vi "mmWave Test Main.vi"() -> ()   [LabVIEW 2019]
doc: "Simple Qued Message Handler type of state machine.\nAlways use this template if the VI is a UI used by a user and it is more complex than a dialog.\n(Unless you're usig something more advanced like Actor Framework)\n\nBolder Software LLC"
uses:
  Support/MessageAPI/RunTest.ctl
  Classes/aparCfg/aparCfg.lvclass
  Classes/Sequence/Sequence.lvclass
  Classes/ExecutionControls/ExecutionControls.lvclass
  Classes/ExecutionStatus/ExecutionStatus.lvclass
  Classes/UI MotionStatus/UI MotionStatus.lvclass
  Classes/SendMessage/SendMessage.lvclass
  Classes/UI ExecutionCtrls/UI ExecutionCtrls.lvclass
  Classes/UI MotionStatus/MotionStatusLEDCtrlRefs.ctl
  Classes/UI MotionStatus/PositonIndicatorsCtrlRefs.ctl
  Classes/UI ExecutionCtrls/MotionExecutionCtrlRefs.ctl
  Classes/UI ExecutionCtrls/mmWaveMotionCrtlRefs.ctl
  Classes/ExecutionControls/ExecutionCtrlRefs.ctl
  Classes/Datalog/DatalogSubvis/SearchableTag.ctl
  Classes/Sequence/SequenceSubvis/RF Direction.ctl
  Classes/Sequence/SequenceSubvis/PolarizationSelect.ctl
  APARMainSubvis/VXM Public API/singleAxisMoveDef.ctl
  APARMainSubvis/VXM Public API/mmWaveAxis.ctl
  Support/MessageQue/MessageQue.lvlib
  Support/UserEvent-ExitEventLoop/UserEvent-ExitEventLoop.lvlib
  Classes/VXMCfg/VXMCfg.lvclass
  Classes/Datalog/DataLog.lvclass
panel:
  out "UIM EventCode":i32
  out "UIM Numeric":dbl
  out "RT2 moving":bool
  out "RT1 moving":bool
  out "BS4 moving":bool
  out "RT2":sgl caption="RT 2, degrees" format="%.2f"
  out "RT1":sgl caption="RT1, degrees" format="%.2f"
  out "BS4":sgl caption="BS 4, mm" format="%.2f"
  in  "Module, 0-63":dbl min=0.0 max=63.0 step=1.0
  out "Temperature, °C":dbl format="%.1g"
  in  "ac read temp":bool
  in  "ac reset":bool
  in  "One Sweep":bool
  in  "Stop Motion":bool
  out "SubSystem 3":bool
  out "SubSystem 2":bool
  in  "FindHomeAll":bool
  in  "Raster Test Sequence Start":bool
  in  "P&M Test Sequence Start":bool
  in  "Run P&M Test":T1
  in  "Polarization":u16(ring) items=["Vertical", "Horizontal"]
  in  "Move to Pos.":bool
  in  "Position":i32=1 caption="Antenna\nPosition" min=0 max=63 step=1
  in  "SeqPanel":bool
  in  "Data File Name":string
  in  "Merge Results":bool
  in  "Merge File and Path":path
  out "Antenna/Raster\nPosition":string
  out "SubSystem 1":bool
  out "RT3 moving":bool
  out "BS3 moving":bool
  out "BS2 moving":bool
  out "BS1 moving":bool
  out "RT3":sgl caption="RT 3, degrees" format="%.2f"
  out "BS3":sgl caption="BS3, mm" format="%.2f"
  out "BS2":sgl caption="BS 2, mm" format="%.2f"
  out "BS1":sgl caption="BS1, mm" format="%.2f"
  in  "Tab":T2(tab)
  in  "Run mode 2":bool
  in  "Run mode 1":bool
  in  "Decimate Update":i32=1
  out "Agilent N5222A Traces":T3(graph)
  out "Progress":u8(slide) scale=0.0..100.0
  out "Sequence Status":string
  in  "ConfigPanel":bool
  in  "Stop":bool
  in  "Run Mode 3":bool
  in  "Pause":bool
  in  "AO Board 2 voltages":dbl[](array[numeric])
  in  "AO Board 1 voltages":dbl[](array[numeric])
  in  "ac d cmd":bool
  in  "RT2 Home Button":bool
  in  "RT2 Jog Neg.":bool
  in  "RT2 Jog Pos.":bool
  in  "Set RT2 Position, Deg.":dbl format="%.4f"
  in  "BS4 Home Button":bool
  in  "BS4 Jog Neg.":bool
  in  "BS4 Jog Pos.":bool
  in  "Set BS4 Position, mm":dbl format="%.4f"
  in  "BS3 Home Button":bool
  in  "BS3 Jog Neg.":bool
  in  "BS3 Jog Pos.":bool
  in  "Set BS3 Position, mm":dbl format="%.4f"
  in  "setHomeSS2":bool
  in  "setHomeSS1":bool
  in  "T Home Button":bool
  in  "T Jog Neg.":bool
  in  "T Jog Pos.":bool
  in  "Set RT3 Position, Deg.":dbl format="%.4f"
  in  "Z Home Button":bool
  in  "Z Jog Neg.":bool
  in  "Z Jog Pos.":bool
  in  "Set RT1 Position, Deg":dbl format="%.4f"
  in  "Y Home Button":bool
  in  "Y Jog Neg.":bool
  in  "Y Jog Pos.":bool
  in  "Set BS2 Position, mm":dbl format="%.4f"
  in  "X Home Button":bool
  in  "X Jog Neg.":bool
  in  "X Jog Pos.":bool
  in  "Set BS1 Position, mm":dbl format="%.4f"
  in  "HomeAll":bool
  in  "MoveAllAbsolute":bool
  in  "Generate \"DAQ\" Loop TestError":bool
  in  "test error":errorcluster
  in  "Generate \"Main\" Loop TestError":bool
  out "i event":i32=6 caption="ievent"
  out "Command":string
  out "i main":i32=6
  # "Park and Measure Positions"
  # "<< make subsyst 1, add button for subsyst 2"
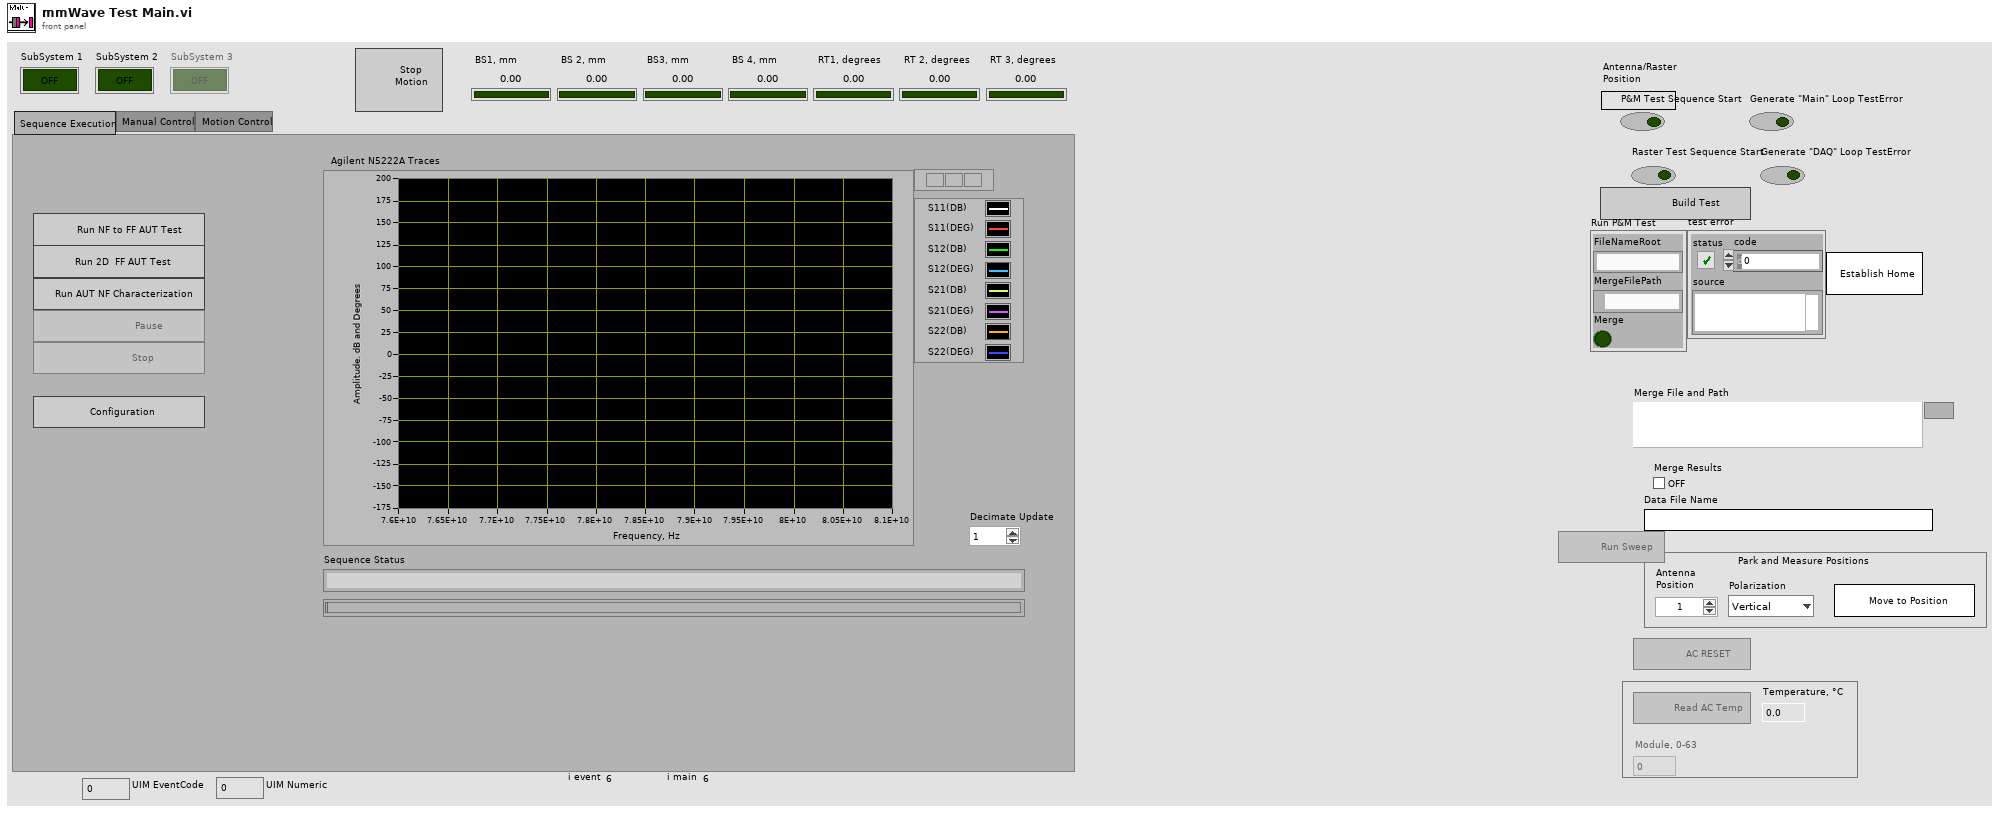
[diagram p1: front panel]
types:
  T1 = typedef "RunTest.ctl" = cluster{"FileNameRoot":string, "MergeFilePath":path, "Merge":bool}
  T2 = enum32{"Sequence Execution", "Manual Control", "Motion Control"}
  T3 = cluster{"array type (2D Dbl)":dbl[], "array type (2D Dbl)":dbl[]}[]
  T4 = cluster{"aparCfg":refnum<class "aparCfg.lvclass">, "Sequence":refnum<class "Sequence.lvclass">, "ExecCtrls":refnum<class "ExecutionControls.lvclass">, "ExecStatus":refnum<class "ExecutionStatus.lvclass">, "graph":i32, "MotionStatus":refnum<class "UI MotionStatus.lvclass">, "SendUIMsg":refnum<class "SendMessage.lvclass">, "MotionExecCtrls":refnum<class "UI ExecutionCtrls.lvclass">}
  T5 = typedef "MultipleMessageQues vxm.ctl" = cluster{"Main que":T6, "Error que":T6, "VXM Svc que":T6, "Listener que":T6, "VXM ACK que":T6, "DAQ que":T6, "Alignment que":T6}
  T6 = typedef "MessageQue.lvlib/MessageQue.ctl" = refnum<queue>
  T7 = typedef "DataLog.lvclass/SearchableTag.ctl" = cluster{"Module, 0-63":i32, "RF Direction Tx0":T8, "Polarization, V0 H1":T9, "AO-64 Array":dbl[]}
  T8 = typedef "RF Direction.ctl" = enum16{"Tx - RF In", "Rx - RF Out"}
  T9 = typedef "PolarizationSelect.ctl" = enum16{"Vertical", "Horizontal"}
  T10 = typedef "mmWaveAxis.ctl" = string
  T11 = typedef "singleAxisMoveDef.ctl" = cluster{"mmWave Axis":T10, "eng. value":dbl}
  T12 = cluster{"Move Type":string, "Positions":T11[], "Position (Antenna or Raster)":i32, "Polarization":u16}
  T13 = typedef "MotionExecutionCtrlRefs.ctl" = cluster{"MoveAllAbsolute":refnum<vi>, "Move to Pos.":refnum<vi>, "HomeAll":refnum<vi>, "FindHomeAll":refnum<vi>, "X Jog Pos.":refnum<vi>, "X Jog Neg.":refnum<vi>, "Y Jog Pos.":refnum<vi>, "Y Jog Neg. ":refnum<vi>, "Z Jog Pos.":refnum<vi>, "Z Jog Neg.":refnum<vi>, "T Jog Pos.":refnum<vi>, "T Jog Neg.":refnum<vi>, "X Home Button":refnum<vi>, "Y Home Button":refnum<vi>, "Z Home Button":refnum<vi>, "T Home Button":refnum<vi>}
  T14 = typedef "PositonIndicatorsCtrlRefs.ctl" = cluster{"BS1":refnum<vi>, "BS2":refnum<vi>, "BS3":refnum<vi>, "BS4":refnum<vi>, "RT3":refnum<vi>, "RT2":refnum<vi>, "RT1":refnum<vi>}
  T15 = typedef "MotionStatusLEDCtrlRefs.ctl" = cluster{"BS1":refnum<vi>, "BS2":refnum<vi>, "BS3":refnum<vi>, "BS4":refnum<vi>, "RT1":refnum<vi>, "RT2":refnum<vi>, "RT3":refnum<vi>}
  T16 = typedef "mmWaveMotionCrtlRefs.ctl" = cluster{"BS3 Jog Neg. 2":refnum<vi>, "BS3 Jog Pos. 2":refnum<vi>, "BS3 Home Button 2":refnum<vi>, "BS4 Jog Neg. 2":refnum<vi>, "BS4 Jog Pos. 2":refnum<vi>, "BS4 Home Button 2":refnum<vi>, "RT2 Jog Neg. 2":refnum<vi>, "RT2 Jog Pos. 2":refnum<vi>, "RT2 Home Button 2":refnum<vi>}
  T17 = typedef "ExecutionCtrlRefs.ctl" = cluster{"Tab":refnum<vi>, "BuildSeqDlg":refnum<vi>, "Run":refnum<vi>, "Pause":refnum<vi>, "Stop":refnum<vi>, "ConfigPanel":refnum<vi>, "SeqStatus":refnum<vi>, "Run raster":refnum<vi>}
  T18 = cluster{"mmWave Names":string[], "Positions this subsystem":dbl[]}
  T19 = typedef "seqConfig.ctl" = cluster{"TempXMLFilePath":path, "Motion":bool}
  T20 = typedef "ACConfig.ctl" = cluster{"Board 1 alias":string, "Board 1 Enable":bool, "Board 2 alias":string, "Board 2 Enable":bool}
  T21 = typedef "N5222AConfig.ctl" = cluster{"ResourceName":string, "Enable":bool, "Channel":i32, "CalFileName":string, "MeasName":string, "TempDatFile":string, "Power, dBm":dbl, "NumPoints":i32, "Start Freq, Hz":dbl, "Stop Freq, Hz":dbl, "NumAverages":i32, "Sweep Type":i32, "IF Bandwidth":dbl}
  T22 = typedef "Mode1TestProperties.ctl" = cluster{"Probe Horizontal Polarization":bool, "Probe Vertical Polarization":bool, "Data File Name":string, "RF In/Out of antenna":T8, "Raster XY Points":cluster{"X mm":dbl, "Y mm":dbl}[]}
  T23 = typedef "Mode2TestProperties.ctl" = cluster{"Probe Horizontal Polarization":bool, "Probe Vertical Polarization":bool, "Upload TR Module file":path, "Data File Name":string, "RF In/Out of antenna":T8, "RT3 Positions, degrees":dbl[]}
  T24 = typedef "Mode3TestProperties.ctl" = cluster{"Probe Horizontal Polarization":bool, "Probe Vertical Polarization":bool, "Upload TR Module file":path, "Data File Name":string, "RF In/Out of antenna":T8}
  T25 = typedef "UIMessage.ctl" = cluster{"EventCode":i32, "Numeric":dbl, "String":string, "Variant":variant}
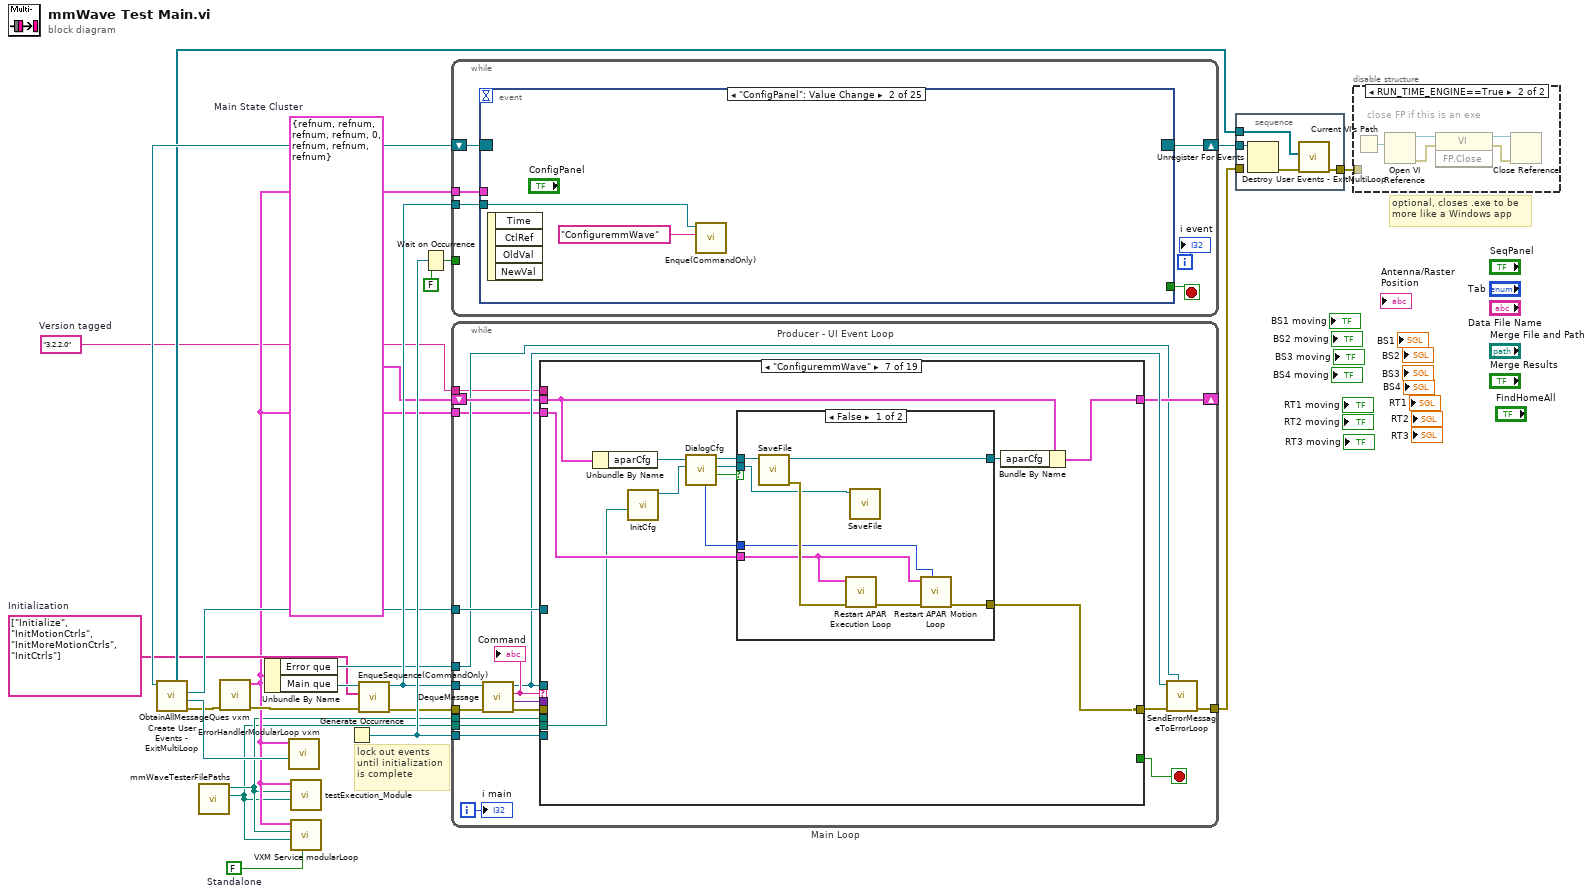
[diagram p0: block diagram]
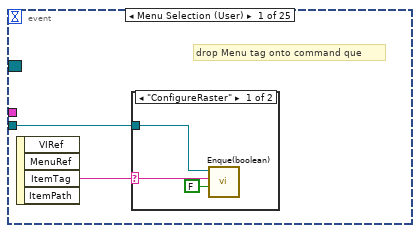
[diagram p3: hidden frame]
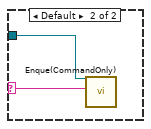
[diagram p4: hidden frame]
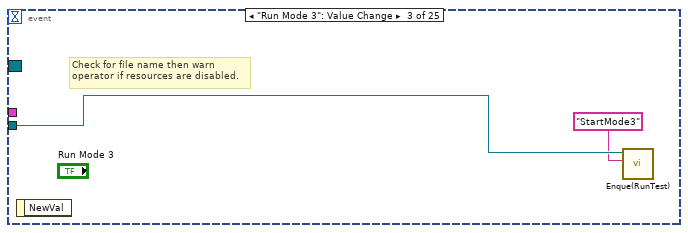
[diagram p5: hidden frame]
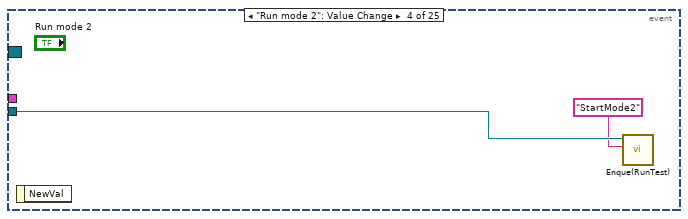
[diagram p6: hidden frame]
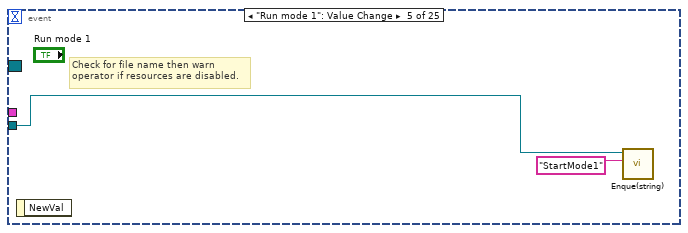
[diagram p7: hidden frame]
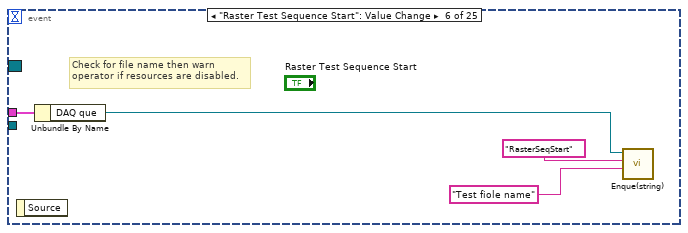
[diagram p8: hidden frame]
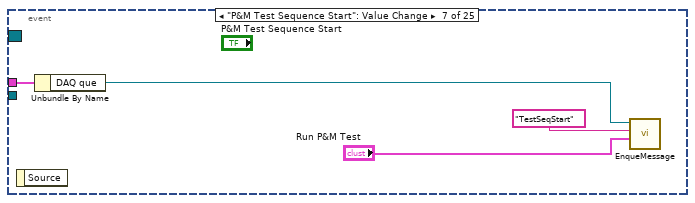
[diagram p9: hidden frame]
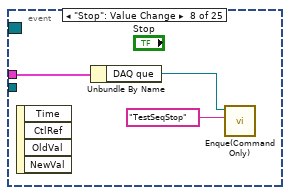
[diagram p10: hidden frame]
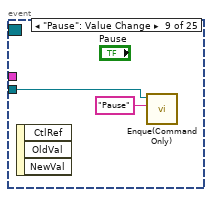
[diagram p11: hidden frame]
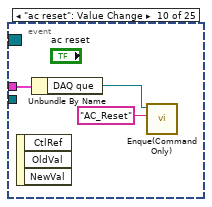
[diagram p12: hidden frame]
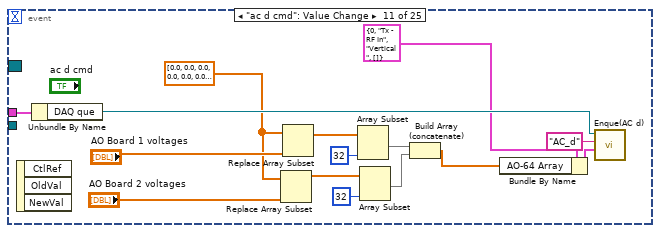
[diagram p13: hidden frame]
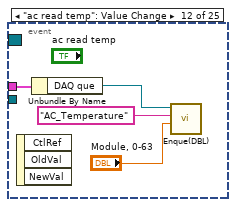
[diagram p14: hidden frame]
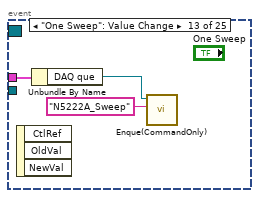
[diagram p15: hidden frame]
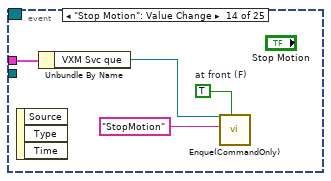
[diagram p16: hidden frame]
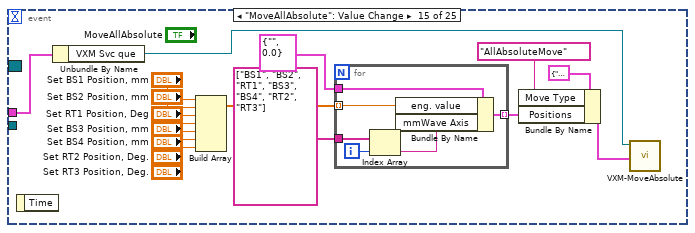
[diagram p17: hidden frame]
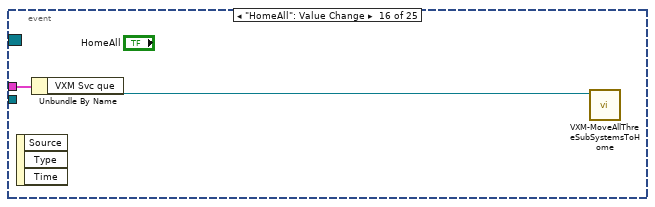
[diagram p18: hidden frame]
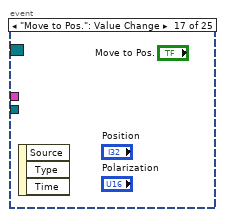
[diagram p19: hidden frame]
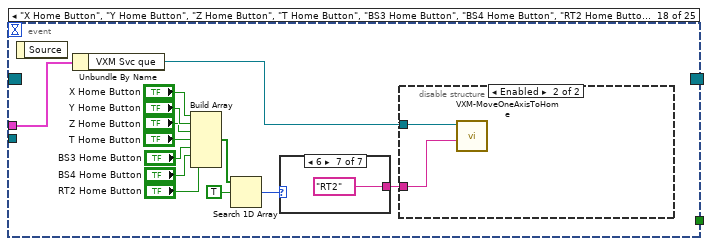
[diagram p20: hidden frame]
diagram:
  w2 = "3.2.2.0"  # Version tagged
  w3 = FALSE  # Standalone
  w9 = string[] ["Initialize", "InitMotionCtrls", "InitMoreMotionCtrls", "InitCtrls"]  # Initialization
  w15 = T4 {"aparCfg"=refnum, "Sequence"=refnum, "ExecCtrls"=refnum, "ExecStatus"=refnum, "graph"=0, "MotionStatus"=refnum, "SendUIMsg"=refnum, "MotionExecCtrls"=refnum}  # Main State Cluster
  # "lock out events\nuntil initialization\nis complete"
  # "optional, closes .exe to be \nmore like a Windows app"
  n1 = call "Create User Events - ExitMultiLoop.vi"() -> ("error out"=w7:errorcluster, "ExitALLLoops event out"=w8:refnum<user-event>, "ExitEventLoop event out"=w10:refnum<user-event>, "Events Registration Refnum"=w18:refnum<event-registration>, "user event array"=w11:refnum<user-event>[])  [unwired: 7 in]
  n2 = call "mmWaveTesterFilePaths.vi"() -> ("Config File Path Motion"=w1:path, "Config File Path"=w4:path)  [unwired: 6 in, 4 out]
  n3 = call "ObtainAllMessageQues vxm.vi"("error in"=w7) -> ("error out"=w6:errorcluster, "MessageQues"=w5:T5)  [unwired: 9 in]
  n4 = Unbundle By Name(w5) -> ("Error que"=w12:T6, "Main que"=w14:T6)
  n5 = call "ErrorHandlerModularLoop vxm.vi"("exit event source"=w8, "MessageQues"=w5) -> ()  [unwired: 9 in, 1 out]
  n6 = call "testExecution_Module.vi"("Motion Cfg File path"=w1, "Cfg File path"=w4, "MessageQues"=w5) -> ()  [unwired: 9 in]
  n7 = call "VXM Service modularLoop.vi"("Standalone"=w3, "Motion Cfg File path"=w1, "Cfg File path"=w4, "MessageQues"=w5) -> ()  [unwired: 8 in]
  n8 = Generate Occurrence() -> (w23:refnum<k4>)
  n9 = call "EnqueSequence(CommandOnly).vi"("error in"=w6, "Message Commands"=w9, "Message que"=w14) -> ("error out"=w20:errorcluster, "Message que out"=w19:T6)  [unwired: 7 in]
  n10 = Wait on Occurrence(1:FALSE ("ignore previous (T)"), 2:w23) -> (0:w17:bool)  [unwired: 1 in]
  n11 = while "Producer - UI Event Loop" {
    shift-right: [w25] -> w22
    shift-left: w18 -> [w26]
    tunnel: w19 -> [w28]
    tunnel: w17 -> [_]
    tunnel: w5 -> [w24]
    i -> [w29]
    stop <- w27 stop-if-true
    n12 = event shown="[1] \"ConfigPanel\": Value Change" {
      selector: w26 -> [_ _ _ _ _ _ _ _ _ _ _ _ _ _ _ _ _ _ _ _ _ _ _ _ _]
      dyn-events: [_ _ _ _ _ _ _ _ _ _ _ _ _ _ _ _ _ _ _ _ _ _ _ _ _] -> w25
      timeout: _ -> [_ _ _ _ _ _ _ _ _ _ _ _ _ _ _ _ _ _ _ _ _ _ _ _ _]
      tunnel: w28 -> [w31 w38 w40 w42 w43 _ _ _ w57 _ _ _ _ _ _ _ _ _ _ _ _ w208 w216 _ _]
      tunnel: [_ _ _ _ _ _ _ _ _ _ _ _ _ _ _ _ _ _ _ _ _ _ _ _ TRUE ("Discard?")] -> w27
      tunnel: w24 -> [_ _ _ _ _ w47 w52 w54 _ w59 w74 w78 w81 w83 w102 w110 _ w117 w147 w176 w200 w211 w214 w222 _]
      event Menu Selection (User) {
        # "drop Menu tag onto command que"
        n13 = event-data() -> ("ItemTag"=w30:string)  [unwired: 1 in, 3 out]
        n14 = case shown="\"ConfigureRaster\"" w30 {
          selector: w30 -> [w32 w35]
          tunnel: w31 -> [w34 w36]
          frame "ConfigureRaster" {
            n15 = call "Enque(boolean).vi"("Message Payload  Boolean"=FALSE, "Message Command"=w32, "Message que"=w34) -> ()  [unwired: 7 in, 2 out]
          }
          frame Default {
            n16 = call "Enque(CommandOnly).vi"("Message Command"=w35, "Message que"=w36) -> ()  [unwired: 8 in, 2 out]
          }
        }
      }
      event "ConfigPanel": Value Change {
        n17 = event-data() -> ()  [unwired: 1 in, 4 out]
        n18 = call "Enque(CommandOnly).vi"("Message Command"="ConfiguremmWave", "Message que"=w38) -> ()  [unwired: 8 in, 2 out]
      }
      event "Run Mode 3": Value Change {
        # "Check for file name then warn\noperator if resources are disabled."
        n19 = event-data() -> ()  [unwired: 1 in, 1 out]
        n20 = call "Enque(RunTest).vi"("Message Command"="StartMode3", "Message que"=w40) -> ()  [unwired: 8 in, 2 out]
      }
      event "Run mode 2": Value Change {
        n21 = event-data() -> ()  [unwired: 1 in, 1 out]
        n22 = call "Enque(RunTest).vi"("Message Command"="StartMode2", "Message que"=w42) -> ()  [unwired: 8 in, 2 out]
      }
      event "Run mode 1": Value Change {
        # "Check for file name then warn\noperator if resources are disabled."
        n23 = event-data() -> ()  [unwired: 1 in, 1 out]
        n24 = call "Enque(string).vi"("Message Command"="StartMode1", "Message que"=w43) -> ()  [unwired: 8 in, 2 out]
      }
      event "Raster Test Sequence Start": Value Change {
        # "Check for file name then warn\noperator if resources are disabled."
        n25 = event-data() -> ()  [unwired: 1 in, 1 out]
        n26 = Unbundle By Name(w47) -> ("DAQ que"=w46:T6)
        n27 = call "Enque(string).vi"("Message Payload string"="Test fiole name", "Message Command"="RasterSeqStart", "Message que"=w46) -> ()  [unwired: 7 in, 2 out]
      }
      event "P&M Test Sequence Start": Value Change {
        n28 = event-data() -> ()  [unwired: 1 in, 1 out]
        n29 = Unbundle By Name(w52) -> ("DAQ que"=w51:T6)
        n30 = call "EnqueMessage.vi"("Message Payload"="Run P&M Test", "Message Command"="TestSeqStart", "Message que"=w51) -> ()  [unwired: 7 in, 2 out]
      }
      event "Stop": Value Change {
        n31 = event-data() -> ()  [unwired: 1 in, 4 out]
        n32 = Unbundle By Name(w54) -> ("DAQ que"=w53:T6)
        n33 = call "Enque(CommandOnly).vi"("Message Command"="TestSeqStop", "Message que"=w53) -> ()  [unwired: 8 in, 2 out]
      }
      event "Pause": Value Change {
        n34 = event-data() -> ()  [unwired: 1 in, 3 out]
        n35 = call "Enque(CommandOnly).vi"("Message Command"="Pause", "Message que"=w57) -> ()  [unwired: 8 in, 2 out]
      }
      event "ac reset": Value Change {
        n36 = event-data() -> ()  [unwired: 1 in, 3 out]
        n37 = Unbundle By Name(w59) -> ("DAQ que"=w58:T6)
        n38 = call "Enque(CommandOnly).vi"("Message Command"="AC_Reset", "Message que"=w58) -> ()  [unwired: 8 in, 2 out]
      }
      event "ac d cmd": Value Change {
        w71 = dbl[] [0.0, 0.0, 0.0, 0.0, 0.0, 0.0, 0.0, 0.0, 0.0, 0.0, 0.0, 0.0, 0.0, 0.0, 0.0, 0.0, 0.0, 0.0, 0.0, 0.0, 0.0, 0.0, 0.0, 0.0, 0.0, 0.0, 0.0, 0.0, 0.0, 0.0, 0.0, 0.0] ("AO Board 1 voltages")
        n39 = event-data() -> ()  [unwired: 1 in, 3 out]
        n40 = Unbundle By Name(w74) -> ("DAQ que"=w73:T6)
        n41 = Replace Array Subset(array=w71, new element="AO Board 2 voltages") -> (w66:dbl[])  [unwired: 1 in]
        n42 = Replace Array Subset(array=w71, new element="AO Board 1 voltages") -> (w68:dbl[])  [unwired: 1 in]
        n43 = Array Subset(array=w68, length=32) -> (w65:dbl[])  [unwired: 1 in]
        n44 = Array Subset(array=w66, length=32) -> (w64:dbl[])  [unwired: 1 in]
        n45 = Build Array (concatenate)(w65, w64) -> (w61:dbl[])
        n46 = Bundle By Name(cluster=T7 {"Module, 0-63"=0, "RF Direction Tx0"=enum."Tx - RF In", "Polarization, V0 H1"=enum."Vertical", "AO-64 Array"=[]} ("d Cmd Payload"), "AO-64 Array"=w61) -> (w62:T7)
        n47 = call "Enque(AC d).vi"("d Cmd Payload"=w62, "Message Command"="AC_d", "Message que"=w73) -> ()  [unwired: 7 in, 2 out]
      }
      event "ac read temp": Value Change {
        n48 = event-data() -> ()  [unwired: 1 in, 3 out]
        n49 = Unbundle By Name(w78) -> ("DAQ que"=w77:T6)
        n50 = call "Enque(DBL).vi"("Message Payload DBL Numeric"="Module, 0-63", "Message Command"="AC_Temperature", "Message que"=w77) -> ()  [unwired: 7 in, 2 out]
      }
      event "One Sweep": Value Change {
        n51 = event-data() -> ()  [unwired: 1 in, 3 out]
        n52 = Unbundle By Name(w81) -> ("DAQ que"=w80:T6)
        n53 = call "Enque(CommandOnly).vi"("Message Command"="N5222A_Sweep", "Message que"=w80) -> ()  [unwired: 8 in, 2 out]
      }
      event "Stop Motion": Value Change {
        w86 = TRUE  # at front (F)
        n54 = event-data() -> ()  [unwired: 1 in, 3 out]
        n55 = Unbundle By Name(w83) -> ("VXM Svc que"=w84:T6)
        n56 = call "Enque(CommandOnly).vi"("at front (F)"=w86, "Message Command"="StopMotion", "Message que"=w84) -> ()  [unwired: 7 in, 2 out]
      }
      event "MoveAllAbsolute": Value Change {
        n57 = event-data() -> ()  [unwired: 1 in, 1 out]
        n58 = Unbundle By Name(w102) -> ("VXM Svc que"=w101:T6)
        n59 = Build Array("Set BS1 Position, mm", "Set BS2 Position, mm", "Set RT1 Position, Deg", "Set BS3 Position, mm", "Set BS4 Position, mm", "Set RT2 Position, Deg.", "Set RT3 Position, Deg.") -> (w89:dbl[])
        n60 = for {
          tunnel: T11 {"mmWave Axis"="", "eng. value"=0.0} ("Move") -> [w108]
          tunnel: w89 -> [w107] mode=indexing
          tunnel: [w106] -> w88 mode=indexing
          tunnel: T10[] ["BS1", "BS2", "RT1", "BS3", "BS4", "RT2", "RT3"] -> [w104]
          i -> [w105]
          n61 = Index Array(array=w104, index=w105) -> (element=w103:T10)
          n62 = Bundle By Name(cluster=w108, "eng. value"=w107, "mmWave Axis"=w103) -> (w106:T11)
        }
        n63 = Bundle By Name(cluster=T12 {"Move Type"="AllAbsoluteMove", "Positions"=[], "Position (Antenna or Raster)"=0, "Polarization"=1} ("Move-Abs"), "Move Type"="AllAbsoluteMove", "Positions"=w88) -> (w99:T12)
        n64 = call "VXM-MoveAbsolute.vi"("Move-Abs"=w99, "Message que"=w101) -> ()  [unwired: 9 in, 1 out]
      }
      event "HomeAll": Value Change {
        n65 = event-data() -> ()  [unwired: 1 in, 3 out]
        n66 = Unbundle By Name(w110) -> ("VXM Svc que"=w109:T6)
        n67 = call "VXM-MoveAllThreeSubSystemsToHome.vi"("Message que"=w109) -> ()  [unwired: 10 in, 1 out]
      }
      event "Move to Pos.": Value Change {
        n68 = event-data() -> ()  [unwired: 1 in, 3 out]
      }
      event "X Home Button", "Y Home Button", "Z Home Button", "T Home Button", "BS3 Home Button", "BS4 Home Button", "RT2 Home Button": Value Change {
        n69 = event-data() -> ()  [unwired: 1 in, 1 out]
        n70 = Unbundle By Name(w117) -> ("VXM Svc que"=w114:T6)
        n71 = Build Array("X Home Button", "Y Home Button", "Z Home Button", "T Home Button", "BS3 Home Button", "BS4 Home Button", "RT2 Home Button") -> (w122:bool[])
        n72 = Search 1D Array(1D array=w122, element=TRUE) -> (index of element=w116:i32)  [unwired: 1 in]
        n73 = case shown="6" w116 {
          tunnel: [T10 "BS1" ("mmWave Axis") T10 "BS2" ("mmWave Axis") T10 "RT1" ("mmWave Axis") T10 "RT3" ("mmWave Axis") T10 "BS3" ("mmWave Axis") T10 "BS4" ("mmWave Axis") T10 "RT2" ("mmWave Axis")] -> w115
          frame 0, Default {
          }
          frame 1 {
          }
          frame 2 {
          }
          frame 3 {
          }
          frame 4 {
          }
          frame 5 {
          }
          frame 6 {
          }
        }
        n74 = disable-structure shown="Enabled" {
          disable-tunnel: w115 -> [w125 w127]
          disable-tunnel: w114 -> [w124 w128]
          frame Disabled {
            n75 = call "EnqueMessage.vi"("Message Payload"=w125, "Message Command"="StartOneAxisMoveToHome", "Message que"=w124) -> ()  [unwired: 7 in, 2 out]
          }
          frame Enabled {
            n76 = call "VXM-MoveOneAxisToHome.vi"("mmWave Axis to home"=w127, "Message que"=w128) -> ()  [unwired: 9 in, 1 out]
          }
        }
      }
      event "X Jog Pos.", "X Jog Neg.", "Y Jog Pos.", "Y Jog Neg.", "Z Jog Pos.", "Z Jog Neg.", "T Jog Pos.", "T Jog Neg.": Value Change {
        n77 = event-data() -> ()  [unwired: 1 in, 1 out]
        n78 = Unbundle By Name(w147) -> ("VXM Svc que"=w137:T6)
        n79 = Build Array("X Jog Pos.", "X Jog Neg.", "Y Jog Pos.", "Y Jog Neg.", "Z Jog Pos.", "Z Jog Neg.", "T Jog Pos.", "T Jog Neg.") -> (w148:bool[])
        n80 = Search 1D Array(1D array=w148, element=TRUE) -> (index of element=w150:i32)  [unwired: 1 in]
        n81 = case shown="0, Default" w150 {
          tunnel: [T10 "BS1" ("mmWave Axis") T10 "BS1" ("mmWave Axis") T10 "BS2" ("mmWave Axis") T10 "BS2" ("mmWave Axis") T10 "RT1" ("mmWave Axis") T10 "RT1" ("mmWave Axis") T10 "RT3" ("mmWave Axis") T10 "RT3" ("mmWave Axis")] -> w138
          tunnel: [1 -1 1 -1 1 -1 1 -1] -> w136
          frame 0, Default {
            # "Axis, direction"
          }
          frame 1 {
            # "Axis, direction"
          }
          frame 2 {
            # "Axis, direction"
          }
          frame 3 {
            # "Axis, direction"
          }
          frame 4 {
            # "Axis, direction"
          }
          frame 5 {
            # "Axis, direction"
          }
          frame 6 {
            # "Axis, direction"
          }
          frame 7 {
            # "Axis, direction"
          }
        }
        n82 = call "VXM-Jog.vi"("Direction"=w136, "mmWave Axis"=w138, "Message que"=w137) -> ()  [unwired: 8 in, 1 out]
      }
      event "BS3 Jog Pos.", "BS3 Jog Neg.", "RT2 Jog Pos.", "RT2 Jog Neg.", "BS4 Jog Pos.", "BS4 Jog Neg.": Value Change {
        n83 = event-data() -> ()  [unwired: 1 in, 1 out]
        n84 = Unbundle By Name(w176) -> ("VXM Svc que"=w174:T6)
        n85 = Build Array("BS3 Jog Pos.", "BS3 Jog Neg.", "RT2 Jog Pos.", "RT2 Jog Neg.", "BS4 Jog Pos.", "BS4 Jog Neg.") -> (w177:bool[])
        n86 = Search 1D Array(1D array=w177, element=TRUE) -> (index of element=w179:i32)  [unwired: 1 in]
        n87 = case shown="5" w179 {
          tunnel: [T10 "BS3" ("mmWave Axis") T10 "BS3" ("mmWave Axis") T10 "RT2" ("mmWave Axis") T10 "RT2" ("mmWave Axis") T10 "BS4" ("mmWave Axis") T10 "BS4" ("mmWave Axis") T10 "RT3" ("mmWave Axis") T10 "RT3" ("mmWave Axis")] -> w175
          tunnel: [1 -1 1 -1 1 -1 1 -1] -> w173
          frame 0, Default {
            # "Axis, direction"
          }
          frame 1 {
            # "Axis, direction"
          }
          frame 2 {
            # "Axis, direction"
          }
          frame 3 {
            # "Axis, direction"
          }
          frame 4 {
            # "Axis, direction"
          }
          frame 5 {
            # "Axis, direction"
          }
          frame 6 {
            # "Axis, direction"
          }
          frame 7 {
            # "Axis, direction"
          }
        }
        n88 = call "VXM-Jog.vi"("Direction"=w173, "mmWave Axis"=w175, "Message que"=w174) -> ()  [unwired: 8 in, 1 out]
      }
      event "setHomeSS1", "setHomeSS2": Value Change {
        w196 = FALSE  # Set Home All Subsystems?
        n89 = event-data() -> ()  [unwired: 1 in, 2 out]
        n90 = Build Array("setHomeSS1", "setHomeSS2") -> (w203:bool[])
        n91 = Unbundle By Name(w200) -> ("VXM Svc que"=w199:T6)
        n92 = Search 1D Array(1D array=w203, element=TRUE) -> (index of element=w198:i32)  [unwired: 1 in]
        n93 = case shown="1" w198 {
          tunnel: [w205 w206] -> w197
          frame 0, Default {
            w205 = 1  # Subsystem 1, 2, 3
          }
          frame 1 {
            w206 = 2  # Subsystem 1, 2, 3
          }
        }
        n94 = call "VXM-SetHome.vi"("Set Home All Axes"=w196, "Subsystem 1, 2, 3"=w197, "Message que"=w199) -> ()  [unwired: 8 in, 1 out]
      }
      event "Generate \"Main\" Loop TestError", "Generate \"DAQ\" Loop TestError": Value Change {
        n95 = event-data() -> ()  [unwired: 1 in, 3 out]
        n96 = Unbundle By Name(w211) -> ("DAQ que"=w209:T6)
        n97 = Select(t=w209, s="Generate \"DAQ\" Loop TestError", f=w208) -> (s? t:f=w207:T6)
        n98 = call "Enque(error).vi"("Message Payload  error cluster"="test error", "Message Command"="GenerateTestError", "Message que"=w207) -> ()  [unwired: 7 in, 2 out]
      }
      event Panel Close? {
        # "Handles x and Ctrl-W"
        n99 = event-data() -> ()  [unwired: 1 in, 2 out]
        n100 = Two Button Dialog(message="Are you sure that you want to exit the program?", 1:"No, Cancel" ("F button name (\"Cancel\")"), 2:"Yes" ("T button name (\"OK\")")) -> (T button?=w215:bool)
        n101 = case shown="True" w215 {
          tunnel: w216 -> [_ _]
          tunnel: w214 -> [_ w221]
          frame False {
          }
          frame True {
            n102 = call "ExitNowAllLoops.vi"("MessageQues"=w221) -> ()  [unwired: 10 in, 1 out]
          }
        }
        n103 = event-data("Discard?"=TRUE) -> ()  [unwired: 1 in, 1 out]
      }
      event User Event {
        n104 = event-data() -> ()  [unwired: 1 in, 3 out]
        n105 = call "ExitNowAllLoops.vi"("MessageQues"=w222) -> ()  [unwired: 10 in, 1 out]
      }
      event User Event {
        n106 = event-data() -> ()  [unwired: 1 in, 3 out]
      }
    }
    "i event" <- w29
  }
  n107 = while "Main Loop" {
    tunnel: w23 -> [w235]
    shift-right: [w230] -> _
    shift-left: w15 -> [w231]
    tunnel: w19 -> [w241]
    tunnel: w20 -> [w240]
    tunnel: w10 -> [w236]
    tunnel: [w229] -> w16
    tunnel: w12 -> [w228]
    tunnel: w5 -> [w227]
    tunnel: w4 -> [w226]
    tunnel: w2 -> [w225]
    tunnel: w1 -> [w224]
    i -> [w242]
    stop <- w234 stop-if-true
    n108 = call "DequeMessage.vi"("error in"=w240, "Message que"=w241) -> ("error out"=w238:errorcluster, "Message Payload"=w237:variant, "Message Command"=w239:string, "Message que out"=w232:T6)  [unwired: 4 in, 2 out]
    "Command" <- w239
    n109 = case shown="\"ConfiguremmWave\"" w239 {
      selector: w239 -> [_ w245 _ _ _ _ _ _ _ _ _ _ _ _ _ _ _ _ _]
      tunnel: w238 -> [_ _ _ _ _ w331 _ w367 _ _ _ w421 w441 _ _ _ _ _ w580]
      tunnel: w232 -> [_ _ _ _ _ _ _ _ _ _ _ _ _ _ _ _ _ _ w578]
      tunnel: w237 -> [_ _ _ _ _ _ _ w366 _ _ _ _ w440 _ _ w570 w573 _ _]
      tunnel: w236 -> [_ _ _ _ _ _ _ _ _ _ _ _ _ _ _ _ _ _ w576]
      tunnel: w235 -> [_ _ _ _ _ w340 _ _ _ _ _ _ _ _ _ _ _ _ _]
      tunnel: [_ _ w250 _ _ w341 w348 w369 w389 w399 w409 w424 w438 _ _ _ w572 _ _] -> w233
      tunnel: [_ _ _ _ _ _ _ _ _ _ _ _ _ _ _ _ _ _ TRUE] -> w234
      tunnel: [w243 w244 w264 w297 w319 w327 w351 w378 w392 w402 w412 w425 w435 w558 w563 w571 w574 w575 w577] -> w230
      tunnel: w231 -> [w243 w244 w257 w298 w320 w328 w352 w379 w392 w402 w412 w426 w436 w558 w563 w571 w574 w575 w577]
      tunnel: w227 -> [_ _ w252 _ _ _ w349 w370 w393 w403 w413 w420 _ _ _ _ _ _ _]
      tunnel: w226 -> [_ _ w262 _ _ _ _ _ _ _ _ _ _ _ _ _ _ _ _]
      tunnel: w225 -> [_ _ _ _ _ _ _ _ _ _ _ _ _ w555 _ _ _ _ _]
      tunnel: w224 -> [_ _ _ _ _ _ w346 _ _ _ _ _ _ _ _ _ _ _ _]
      frame "idle" {
      }
      frame Default {
        # "handles erroneous command strings"
        n110 = Concatenate Strings("WARNING\n" ("message"), w245, " is not a case in this VI" ("message")) -> (w248:string)
        n111 = One Button Dialog(message=w248) -> ()  [unwired: 1 in, 1 out]
      }
      frame "Initialize" {
        w254 = refnum<class "SendMessage.lvclass"> refnum  # SendUIMsg
        # "^ use this to send UI messages\nto the alignment panel"
        # "get exe version Fab style"
        n112 = Unbundle By Name(w252) -> ("Alignment que"=w249:T6)
        n113 = Unbundle By Name(w257) -> ("Sequence"=w256:refnum<class "Sequence.lvclass">)
        n114 = call "InitCfg.vi"("Cfg File path"=w262) -> ("error out"=w261:errorcluster, "aparCfg out"=w263:refnum<class "aparCfg.lvclass">)  [unwired: 9 in]
        n115 = call "ReadAll.vi"("error in (no error)"=w261, "aparCfg in"=w263) -> ("error out"=w260:errorcluster, "aparCfg out"=w258:refnum<class "aparCfg.lvclass">, "SequenceConfig"=w259:T19)  [unwired: 4 in, 3 out]
        n116 = call "LoadSequence.vi"("error in (no error)"=w260, "Sequence Cfg"=w259, "Sequence in"=w256) -> ("error out"=w251:errorcluster, "Sequence out"=w255:refnum<class "Sequence.lvclass">)  [unwired: 7 in]
        n117 = call "RegisterMessageQue.vi"("error in (no error)"=w251, "Message que"=w249, "SendMessage in"=w254) -> ("error out"=w250:errorcluster, "SendMessage out"=w253:refnum<class "SendMessage.lvclass">)  [unwired: 7 in]
        n118 = Bundle By Name(cluster=w257, "aparCfg"=w258, "Sequence"=w255, "SendUIMsg"=w253) -> (w264:T4)
      }
      frame "InitMotionCtrls" {
        w266 = FALSE ("Home Established")
        # "Home indicators"
        # "gather references for indicators and controls separately"
        n119 = control-ref of="BS1 moving"() -> (w278:refnum<vi>)
        n120 = control-ref of="BS2 moving"() -> (w277:refnum<vi>)
        n121 = control-ref of="BS3 moving"() -> (w276:refnum<vi>)
        n122 = control-ref of="BS4 moving"() -> (w275:refnum<vi>)
        n123 = control-ref of="RT1 moving"() -> (w272:refnum<vi>)
        n124 = control-ref of="RT2 moving"() -> (w274:refnum<vi>)
        n125 = control-ref of="RT3 moving"() -> (w273:refnum<vi>)
        n126 = control-ref of="BS1"() -> (w301:refnum<vi>)
        n127 = control-ref of="BS2"() -> (w300:refnum<vi>)
        n128 = control-ref of="BS3"() -> (w299:refnum<vi>)
        n129 = control-ref of="BS4"() -> (w271:refnum<vi>)
        n130 = control-ref of="RT2"() -> (w270:refnum<vi>)
        n131 = control-ref of="RT1"() -> (w269:refnum<vi>)
        n132 = control-ref of="RT3"() -> (w268:refnum<vi>)
        n133 = Bundle By Name(cluster=T14 {"BS1"=refnum, "BS2"=refnum, "BS3"=refnum, "BS4"=refnum, "RT3"=refnum, "RT2"=refnum, "RT1"=refnum} ("PositionIndCtrls"), "BS1"=w301, "BS2"=w300, "BS3"=w299, "BS4"=w271, "RT3"=w270, "RT2"=w269, "RT1"=w268) -> (w279:T14)
        n134 = Bundle By Name(cluster=T15 {"BS1"=refnum, "BS2"=refnum, "BS3"=refnum, "BS4"=refnum, "RT1"=refnum, "RT2"=refnum, "RT3"=refnum} ("MotionStatusCtrls"), "BS1"=w278, "BS2"=w277, "BS3"=w276, "BS4"=w275, "RT1"=w272, "RT2"=w274, "RT3"=w273) -> (w302:T15)
        n135 = call "Init.vi"("PositionIndCtrls"=w279, "MotionStatusCtrls"=w302) -> ("UI MotionStatus out"=w305:refnum<class "UI MotionStatus.lvclass">)  [unwired: 8 in, 1 out]
        n136 = control-ref of="MoveAllAbsolute"() -> (w295:refnum<vi>)
        n137 = control-ref of="Move to Pos."() -> (w294:refnum<vi>)
        n138 = control-ref of="HomeAll"() -> (w293:refnum<vi>)
        n139 = control-ref of="FindHomeAll"() -> (w292:refnum<vi>)
        n140 = control-ref of="X Jog Pos."() -> (w291:refnum<vi>)
        n141 = control-ref of="X Jog Neg."() -> (w290:refnum<vi>)
        n142 = control-ref of="Y Jog Pos."() -> (w289:refnum<vi>)
        n143 = control-ref of="Y Jog Neg."() -> (w288:refnum<vi>)
        n144 = control-ref of="Z Jog Pos."() -> (w287:refnum<vi>)
        n145 = control-ref of="Z Jog Neg."() -> (w286:refnum<vi>)
        n146 = control-ref of="T Jog Pos."() -> (w285:refnum<vi>)
        n147 = control-ref of="T Jog Neg."() -> (w284:refnum<vi>)
        n148 = control-ref of="X Home Button"() -> (w283:refnum<vi>)
        n149 = control-ref of="Y Home Button"() -> (w282:refnum<vi>)
        n150 = control-ref of="Z Home Button"() -> (w281:refnum<vi>)
        n151 = control-ref of="T Home Button"() -> (w280:refnum<vi>)
        n152 = Bundle(cluster=T13 {"MoveAllAbsolute"=refnum, "Move to Pos."=refnum, "HomeAll"=refnum, "FindHomeAll"=refnum, "X Jog Pos."=refnum, "X Jog Neg."=refnum, "Y Jog Pos."=refnum, "Y Jog Neg. "=refnum, "Z Jog Pos."=refnum, "Z Jog Neg."=refnum, "T Jog Pos."=refnum, "T Jog Neg."=refnum, "X Home Button"=refnum, "Y Home Button"=refnum, "Z Home Button"=refnum, "T Home Button"=refnum} ("ExecCtrlRefs"), "MoveAllAbsolute"=w295, "Move to Pos."=w294, "HomeAll"=w293, "FindHomeAll"=w292, "X Jog Pos."=w291, "X Jog Neg."=w290, "Y Jog Pos."=w289, "Y Jog Neg."=w288, "Z Jog Pos."=w287, "Z Jog Neg."=w286, "T Jog Pos."=w285, "T Jog Neg."=w284, "X Home Button"=w283, "Y Home Button"=w282, "Z Home Button"=w281, "T Home Button"=w280) -> (w304:T13)
        n153 = call "Init.vi"("ExecCtrlRefs"=w304) -> ("UI ExecutionCtrls out"=w265:refnum<class "UI ExecutionCtrls.lvclass">)  [unwired: 9 in, 1 out]
        n154 = Bundle By Name(cluster=w298, "MotionStatus"=w305, "MotionExecCtrls"=w265) -> (w297:T4)
        n155 = local write "SubSystem 2"(w266) -> ()
        n156 = local write "SubSystem 3"(w266) -> ()
        n157 = local write "SubSystem 1"(w266) -> ()
      }
      frame "InitMoreMotionCtrls" {
        # "more controls"
        n158 = Unbundle By Name(w320) -> ("MotionExecCtrls"=w306:refnum<class "UI ExecutionCtrls.lvclass">)
        n159 = control-ref of="BS3 Home Button"() -> (w309:refnum<vi>)
        n160 = control-ref of="BS3 Jog Neg."() -> (w308:refnum<vi>)
        n161 = control-ref of="BS3 Jog Pos."() -> (w307:refnum<vi>)
        n162 = control-ref of="BS4 Jog Neg."() -> (w315:refnum<vi>)
        n163 = control-ref of="BS4 Jog Pos."() -> (w314:refnum<vi>)
        n164 = control-ref of="BS4 Home Button"() -> (w313:refnum<vi>)
        n165 = control-ref of="RT2 Jog Neg."() -> (w312:refnum<vi>)
        n166 = control-ref of="RT2 Jog Pos."() -> (w311:refnum<vi>)
        n167 = control-ref of="RT2 Home Button"() -> (w310:refnum<vi>)
        n168 = Bundle By Name(cluster=T16 {"BS3 Jog Neg. 2"=refnum, "BS3 Jog Pos. 2"=refnum, "BS3 Home Button 2"=refnum, "BS4 Jog Neg. 2"=refnum, "BS4 Jog Pos. 2"=refnum, "BS4 Home Button 2"=refnum, "RT2 Jog Neg. 2"=refnum, "RT2 Jog Pos. 2"=refnum, "RT2 Home Button 2"=refnum} ("mmWave motion ctrls"), "BS3 Jog Neg. 2"=w309, "BS3 Jog Pos. 2"=w308, "BS3 Home Button 2"=w307, "BS4 Jog Neg. 2"=w315, "BS4 Jog Pos. 2"=w314, "BS4 Home Button 2"=w313, "RT2 Jog Neg. 2"=w312, "RT2 Jog Pos. 2"=w311, "RT2 Home Button 2"=w310) -> (w316:T16)
        n169 = call "addmmWaveRefnums.vi"("mmWave motion ctrls"=w316, "UI ExecutionCtrls in"=w306) -> ("UI ExecutionCtrls out"=w318:refnum<class "UI ExecutionCtrls.lvclass">)  [unwired: 8 in, 1 out]
        n170 = Bundle By Name(cluster=w320, "MotionExecCtrls"=w318) -> (w319:T4)
      }
      frame "InitCtrls" {
        (unwired) refnum<vi> refnum ("Sequence Status")
        n171 = Unbundle By Name(w328) -> ("ExecCtrls"=w330:refnum<class "ExecutionControls.lvclass">)
        n172 = control-ref of="Tab"() -> (w338:refnum<vi>)
        n173 = control-ref of="Run mode 1"() -> (w321:refnum<vi>)
        n174 = control-ref of="BuildSeqDlg"() -> (w333:refnum<vi>)
        n175 = control-ref of="Run Mode 3"() -> (w334:refnum<vi>)
        n176 = control-ref of="Pause"() -> (w335:refnum<vi>)
        n177 = control-ref of="Stop"() -> (w336:refnum<vi>)
        n178 = control-ref of="ConfigDlg"() -> (w337:refnum<vi>)
        n179 = control-ref of="Sequence Status"() -> (w324:refnum<vi>)
        n180 = local write "Progress"(u8 0 ("Progress")) -> ()
        n181 = Bundle By Name(cluster=T17 {"Tab"=refnum, "BuildSeqDlg"=refnum, "Run"=refnum, "Pause"=refnum, "Stop"=refnum, "ConfigPanel"=refnum, "SeqStatus"=refnum, "Run raster"=refnum} ("output cluster"), "Tab"=w338, "BuildSeqDlg"=w333, "Run"=w334, "Pause"=w335, "Stop"=w336, "ConfigPanel"=w337, "SeqStatus"=w324, "Run raster"=w321) -> (w329:T17)
        n182 = call "Init.vi"("error in (no error)"=w331, "CtrlRefs"=w329, "ExecutionControls in"=w330) -> ("error out"=w332:errorcluster, "ExecutionControls out"=w326:refnum<class "ExecutionControls.lvclass">)  [unwired: 7 in]
        n183 = stacked-sequence {
          tunnel: w332 -> [w342]
          tunnel: [w342] -> w341
          tunnel: w340 -> [w343]
          frame #0 {
            (unwired) "let user events happen now. Make sure nothing goes to the error handler prior to this ocurrance firing, or the VI will be frozen."
            n184 = Set Occurrence(w343) -> ()
          }
        }
        n185 = local write "Decimate Update"(1 ("Decimate Update")) -> ()
        n186 = Bundle By Name(cluster=w328, "ExecCtrls"=w326) -> (w327:T4)
        n187 = property on="Agilent N5222A Traces" class="XYGraph (strict)"("Value"=T3 [] ("Agilent N5222A Traces")) -> ()  [unwired: 2 in, 2 out]
      }
      frame "ConfiguremmWave" {
        n188 = Unbundle By Name(w352) -> ("aparCfg"=w355:refnum<class "aparCfg.lvclass">)
        n189 = call "InitCfg.vi"("Cfg File path"=w346) -> ("VXMCfg out"=w345:refnum<class "VXMCfg.lvclass">)  [unwired: 8 in, 2 out]
        n190 = call "DialogCfg.vi"("VXMCfg in"=w345, "aparCfg in"=w355) -> ("Cancelled?"=w350:bool, "VXMCfg out"=w344:refnum<class "VXMCfg.lvclass">, "aparCfg out"=w354:refnum<class "aparCfg.lvclass">, "Motion Restart"=w347:enum16{"NoOp", "Start", "Stop"})  [unwired: 5 in, 1 out]
        n191 = case shown="False" w350 {
          tunnel: w354 -> [w363 w364]
          tunnel: [w362 w364] -> w353
          tunnel: w349 -> [w357 _]
          tunnel: [w359 _] -> w348
          tunnel: w347 -> [w358 _]
          tunnel: w344 -> [w356 _]
          frame False {
            n192 = call "SaveFile.vi"("aparCfg in"=w363) -> ("error out"=w361:errorcluster, "aparCfg out"=w362:refnum<class "aparCfg.lvclass">)  [unwired: 9 in]
            n193 = call "Restart APAR Execution Loop.vi"("error in"=w361, "MessageQues"=w357) -> ("error out"=w360:errorcluster)  [unwired: 9 in]
            n194 = call "SaveFile.vi"("VXMCfg in"=w356) -> ()  [unwired: 9 in, 2 out]
            n195 = call "Restart APAR Motion Loop.vi"("Motion restart"=w358, "error in"=w360, "MessageQues"=w357) -> ("error out"=w359:errorcluster)  [unwired: 8 in]
          }
          frame True {
          }
        }
        n196 = Bundle By Name(cluster=w352, "aparCfg"=w353) -> (w351:T4)
      }
      frame "StartTestSequence" {
        # "send message to APAR\nExecution Loop to start"
        # "warn if AC or N5222A are disabled"
        # "Check config file"
        n197 = call "ConvertTo(RunTest).vi"("error in"=w367, "Message Payload"=w366) -> ("RunTest"=w365:T1)  [unwired: 8 in, 1 out]
        n198 = Unbundle By Name(w379) -> ("aparCfg"=w377:refnum<class "aparCfg.lvclass">)
        n199 = call "ReadAll.vi"("aparCfg in"=w377) -> ("error out"=w369:errorcluster, "ACConfig"=w375:T20, "N5222A Cfg"=w376:T21, "aparCfg out"=w368:refnum<class "aparCfg.lvclass">)  [unwired: 5 in, 2 out]
        n200 = Unbundle By Name(w375) -> ("Board 2 Enable"=w374:bool)
        n201 = Unbundle By Name(w376) -> ("Enable"=w373:bool)
        n202 = And(x=w373, y=w374) -> (x .and. y?=w371:bool)
        n203 = case shown="False" w371 {
          selector: w371 -> [_ w388]
          tunnel: [w384 w388] -> w372
          frame False {
            n204 = Two Button Dialog(message="One or more instruments are disabled.\n\nSelect the menu Window > Configure APAR Test ... to change this.", 1:"Do Not Start Test" ("F button name (\"Cancel\")"), 2:"Start Test" ("T button name (\"OK\")")) -> (T button?=w384:bool)
          }
          frame True {
          }
        }
        n205 = case shown="True" w372 {
          tunnel: w370 -> [_ w381]
          tunnel: w365 -> [_ w380]
          frame False {
          }
          frame True {
            n206 = Unbundle By Name(w381) -> ("DAQ que"=w382:T6)
            n207 = call "Enque(RunTest).vi"("RunTest"=w380, "Message Command"="TestSeqStart", "Message que"=w382) -> ()  [unwired: 7 in, 2 out]
          }
        }
        n208 = Bundle By Name(cluster=w379, "aparCfg"=w368) -> (w378:T4)
      }
      frame "StartMode1" {
        n209 = call "Mode 1 - NFScanPositionDefinition.vi"() -> ("Cancel = True"=w391:bool, "Mode3TestProperties"=w390:T22)  [unwired: 10 in]
        n210 = case shown="False" w391 {
          tunnel: w393 -> [w398 _]
          tunnel: w390 -> [w395 _]
          tunnel: [w394 _] -> w389
          frame False {
            # "Start a Mode1 test"
            n211 = Unbundle By Name(w398) -> ("DAQ que"=w397:T6)
            n212 = call "EnqueMessage.vi"("Message Payload"=w395, "Message Command"="Mode1Start", "Message que"=w397) -> ("error out"=w394:errorcluster)  [unwired: 7 in, 1 out]
          }
          frame True {
            # "dialog cancelled"
          }
        }
      }
      frame "StartMode2" {
        n213 = call "Mode 2 - 2D FF AUT Test.vi"() -> ("Mode2 Test Properties"=w400:T23, "Cancelled?"=w401:bool)  [unwired: 10 in]
        n214 = case shown="False" w401 {
          tunnel: w403 -> [w408 _]
          tunnel: w400 -> [w405 _]
          tunnel: [w404 _] -> w399
          frame False {
            # "Start a Mode2 test"
            n215 = Unbundle By Name(w408) -> ("DAQ que"=w407:T6)
            n216 = call "EnqueMessage.vi"("Message Payload"=w405, "Message Command"="Mode2Start", "Message que"=w407) -> ("error out"=w404:errorcluster)  [unwired: 7 in, 1 out]
          }
          frame True {
            # "dialog cancelled"
          }
        }
      }
      frame "StartMode3" {
        n217 = call "Mode 3 - AUT NF Characterization.vi"() -> ("Mode3 Test Properties"=w410:T24, "Cancelled?"=w411:bool)  [unwired: 10 in]
        n218 = case shown="False" w411 {
          tunnel: w413 -> [w418 _]
          tunnel: w410 -> [w415 _]
          tunnel: [w414 _] -> w409
          frame False {
            # "Start a Mode3 test"
            n219 = Unbundle By Name(w418) -> ("DAQ que"=w417:T6)
            n220 = call "EnqueMessage.vi"("Message Payload"=w415, "Message Command"="Mode3Start", "Message que"=w417) -> ("error out"=w414:errorcluster)  [unwired: 7 in, 1 out]
          }
          frame True {
            # "dialog cancelled"
          }
        }
      }
      frame "Pause" {
        n221 = Unbundle By Name(w420) -> ("DAQ que"=w419:T6)
        n222 = Unbundle By Name(w426) -> ("ExecCtrls"=w428:refnum<class "ExecutionControls.lvclass">)
        n223 = call "Read ExecutionState.vi"("error in (no error)"=w421, "ExecutionControls in"=w428) -> ("error out"=w423:errorcluster, "Paused = T"=w429:bool, "ExecutionControls out"=w427:refnum<class "ExecutionControls.lvclass">)  [unwired: 6 in, 1 out]
        n224 = Select(t="TestSeqResume" ("Message Command"), s=w429, f="TestSeqPause" ("Message Command")) -> (s? t:f=w422:string)
        n225 = Bundle By Name(cluster=w426, "ExecCtrls"=w427) -> (w425:T4)
        n226 = call "Enque(CommandOnly).vi"("error in"=w423, "Message Command"=w422, "Message que"=w419) -> ("error out"=w424:errorcluster)  [unwired: 7 in, 1 out]
      }
      frame "UIMessage" {
        n227 = call "ConvertTo(UIMessage).vi"("error in"=w441, "Message Payload"=w440) -> ("error out"=w439:errorcluster, "UIMsg"=w437:T25)  [unwired: 8 in]
        n228 = Unbundle By Name(w437) -> ("EventCode"=w432:i32, "Numeric"=w434:dbl, "String"=w433:string)  [unwired: 1 out]
        "UIM Numeric" <- w434
        "UIM EventCode" <- w432
        n229 = case shown="1, Default" w432 {
          tunnel: w433 -> [_ w442]
          frame 10, 11, 104, 106 {
          }
          frame 1, Default {
            n230 = case shown="Default" w442 {
              selector: w442 -> [w443 _]
              frame Default {
                "Sequence Status" <- w443
              }
              frame "" {
              }
            }
          }
        }
        n231 = case shown="10" w432 {
          tunnel: [w444 w446 w453 w458 w464 w470 w474 w476 w486 _ _ _ _ _ _ _ _ _ _] -> w438
          tunnel: w439 -> [w444 w452 w453 w460 w466 w472 w474 w476 w486 _ _ _ _ _ _ _ _ _ _]
          tunnel: w437 -> [_ _ _ _ _ _ _ _ _ _ _ _ _ _ _ w535 _ _ _]
          tunnel: w436 -> [w445 w450 w454 w455 w461 w469 w475 w478 w481 w489 w491 w494 w500 w509 w517 w531 w543 w547 w554]
          tunnel: [w445 w449 w454 w457 w463 w468 w475 w478 w480 w489 w491 w494 w500 w509 w517 w531 w543 w547 w554] -> w435
          tunnel: w434 -> [_ _ _ _ _ _ w473 w477 _ _ _ w492 _ _ _ _ _ w544 w551]
          tunnel: w433 -> [_ _ _ _ _ _ _ _ w485 _ _ _ w497 w507 w516 _ _ w545 w552]
          frame 0, Default {
          }
          frame 3 {
            n232 = Unbundle By Name(w450) -> ("ExecCtrls"=w451:refnum<class "ExecutionControls.lvclass">)
            n233 = call "StartAutoTest.vi"("error in (no error)"=w452, "ExecutionControls in"=w451) -> ("error out"=w446:errorcluster, "ExecutionControls out"=w448:refnum<class "ExecutionControls.lvclass">)  [unwired: 8 in]
            n234 = local write "Progress"(u8 0 ("Progress")) -> ()
            n235 = Bundle By Name(cluster=w450, "ExecCtrls"=w448) -> (w449:T4)
          }
          frame 4 {
            # "Trace"
          }
          frame 5 {
            # "PauseAutoTest"
            n236 = Unbundle By Name(w455) -> ("ExecCtrls"=w459:refnum<class "ExecutionControls.lvclass">)
            n237 = call "PauseAutoTest.vi"("error in (no error)"=w460, "ExecutionControls in"=w459) -> ("error out"=w458:errorcluster, "ExecutionControls out"=w456:refnum<class "ExecutionControls.lvclass">)  [unwired: 8 in]
            n238 = Bundle By Name(cluster=w455, "ExecCtrls"=w456) -> (w457:T4)
          }
          frame 6 {
            # "ResumeAutoTest"
            n239 = Unbundle By Name(w461) -> ("ExecCtrls"=w465:refnum<class "ExecutionControls.lvclass">)
            n240 = call "ResumeAutoTest.vi"("error in (no error)"=w466, "ExecutionControls in"=w465) -> ("error out"=w464:errorcluster, "ExecutionControls out"=w462:refnum<class "ExecutionControls.lvclass">)  [unwired: 8 in]
            n241 = Bundle By Name(cluster=w461, "ExecCtrls"=w462) -> (w463:T4)
          }
          frame 7 {
            # "Sequence compete"
            n242 = Unbundle By Name(w469) -> ("ExecCtrls"=w471:refnum<class "ExecutionControls.lvclass">)
            n243 = call "CompleteAutoTest.vi"("error in (no error)"=w472, "ExecutionControls in"=w471) -> ("error out"=w470:errorcluster, "ExecutionControls out"=w467:refnum<class "ExecutionControls.lvclass">)  [unwired: 8 in]
            n244 = Bundle By Name(cluster=w469, "ExecCtrls"=w467) -> (w468:T4)
          }
          frame 8 {
            "Temperature, °C" <- w473
          }
          frame 9 {
            "Progress" <- w477
          }
          frame 10 {
            # "PNA trace"
            n245 = Unbundle By Name(w481) -> ("graph"=w484:i32)
            n246 = Quotient & Remainder(x=w484, y="Decimate Update") -> (x-y*floor(x/y)=w479:i32)  [unwired: 1 out]
            n247 = Increment(x=w484) -> (x+1=w482:i32)
            n248 = case shown="0" w479 {
              tunnel: w485 -> [_ w488]
              frame 1, Default {
                # "skip update"
              }
              frame 0 {
                n249 = call "UI Message Graph N5222A traces file.vi"("PNA .csv File"=w488) -> ("XY Graph"=→"Agilent N5222A Traces":T3)  [unwired: 10 in]
              }
            }
            n250 = Bundle By Name(cluster=w481, "graph"=w482) -> (w480:T4)
          }
          frame 11 {
            # "noop"
          }
          frame 100 {
            # "100 Motion Started"
            n251 = Unbundle By Name(w491) -> ("MotionExecCtrls"=w490:refnum<class "UI ExecutionCtrls.lvclass">)  [unwired: 2 out]
            n252 = call "StartMotion.vi"("UI ExecutionCtrls in"=w490) -> ()  [unwired: 9 in, 2 out]
          }
          frame 101 {
            # "#deadcode whole case delete"
            # "101 Motion Stopped"
            n253 = Unbundle By Name(w494) -> ("MotionStatus"=w493:refnum<class "UI MotionStatus.lvclass">)  [unwired: 2 out]
            n254 = disable-structure shown="Disabled" {
              disable-tunnel: w493 -> [w496 _]
              disable-tunnel: w492 -> [w495 _]
              frame Disabled {
                n255 = call "StopMotion.vi"("Axis, 1 - 4"=w495, "UI MotionStatus in"=w496) -> ()  [unwired: 8 in, 2 out]
              }
              frame Enabled {
              }
            }
          }
          frame 102 {
            # "#deadcode"
            # "102 Stop Motion command invoked"
            n256 = Unbundle By Name(w500) -> ("MotionExecCtrls"=w498:refnum<class "UI ExecutionCtrls.lvclass">, "MotionStatus"=w499:refnum<class "UI MotionStatus.lvclass">)  [unwired: 1 out]
            n257 = disable-structure shown="Disabled" {
              disable-tunnel: w499 -> [w502 _]
              disable-tunnel: w497 -> [w501 _]
              frame Disabled {
                n258 = Spreadsheet String To Array(delimiter (Tab)=",", format string="%.5f", spreadsheet string=w501, array type (2D Dbl)=dbl[] []) -> (array=w506:dbl[])
                n259 = call "WriteAllPositions.vi"("Positions, mm"=w506, "UI MotionStatus in"=w502) -> ()  [unwired: 8 in, 2 out]
              }
              frame Enabled {
              }
            }
            n260 = call "StopMotion.vi"("UI ExecutionCtrls in"=w498) -> ()  [unwired: 9 in, 2 out]
          }
          frame 103 {
            # "#deadcode"
            # "update all four positions, position only not LEDs"
            n261 = Unbundle By Name(w509) -> ("MotionStatus"=w508:refnum<class "UI MotionStatus.lvclass">)
            n262 = disable-structure shown="Disabled" {
              disable-tunnel: w508 -> [w511 _]
              disable-tunnel: w507 -> [w510 _]
              frame Disabled {
                n263 = Spreadsheet String To Array(delimiter (Tab)=",", format string="%.5f", spreadsheet string=w510, array type (2D Dbl)=dbl[] []) -> (array=w515:dbl[])
                n264 = call "WriteAllPositions.vi"("Positions, mm"=w515, "UI MotionStatus in"=w511) -> ()  [unwired: 8 in, 2 out]
              }
              frame Enabled {
              }
            }
          }
          frame 104 {
            # "#deadcode"
            # "104 update one position"
            n265 = Unbundle By Name(w517) -> ("MotionStatus"=w518:refnum<class "UI MotionStatus.lvclass">)  [unwired: 1 out]
            n266 = disable-structure shown="Disabled" {
              disable-tunnel: w518 -> [w520 _]
              disable-tunnel: w516 -> [w519 _]
              frame Disabled {
                n267 = Spreadsheet String To Array(delimiter (Tab)=",", format string="%.5f", spreadsheet string=w519, array type (2D Dbl)=dbl[] []) -> (array=w524:dbl[])
                n268 = Index Array(array=w524) -> (element #1=w526:dbl, element #2=w525:dbl)  [unwired: 2 in]
                n269 = call "WriteOnePosition.vi"("Axis, 1 - 4"=w526, "Position, counts"=w525, "UI MotionStatus in"=w520) -> ()  [unwired: 7 in, 2 out]
              }
              frame Enabled {
              }
            }
          }
          frame 105 {
            n270 = Unbundle By Name(w531) -> ("MotionStatus"=w530:refnum<class "UI MotionStatus.lvclass">)
            n271 = Unbundle By Name(w535) -> ("Variant"=w533:variant, "Numeric"=w534:dbl)
            n272 = Variant To Data(type=T18 {"mmWave Names"=[], "Positions this subsystem"=[]} ("mmWave names, positions"), Variant=w533) -> (data=w529:T18)  [unwired: 1 in, 1 out]
            n273 = Unbundle By Name(w529) -> ("mmWave Names"=w528:string[], "Positions this subsystem"=w527:dbl[])
            n274 = case shown="1" w534 {
              frame 0, Default {
              }
              frame 1 {
                "SubSystem 1" <- TRUE ("Home Established")
              }
              frame 2 {
                "SubSystem 2" <- TRUE
              }
              frame 3 {
                "SubSystem 3" <- TRUE
              }
            }
            n275 = for {
              tunnel: w530 -> [w538]
              tunnel: w528 -> [w537] mode=indexing
              tunnel: w527 -> [w536] mode=indexing
              n276 = call "WritemmWavePosition.vi"("Axis Position, eng."=w536, "mmWave Axis Name"=w537, "UI MotionStatus in"=w538) -> ()  [unwired: 7 in, 2 out]
            }
          }
          frame 106 {
            # "End of a long/four axis motion"
            n277 = Unbundle By Name(w543) -> ("MotionExecCtrls"=w542:refnum<class "UI ExecutionCtrls.lvclass">)  [unwired: 2 out]
            n278 = call "StopMotion.vi"("UI ExecutionCtrls in"=w542) -> ()  [unwired: 9 in, 2 out]
          }
          frame 1000 {
            # "motion started or stopped, mmWave"
            n279 = Unbundle By Name(w547) -> ("MotionStatus"=w546:refnum<class "UI MotionStatus.lvclass">)
            n280 = call "WritemmWavePosition.vi"("Axis Position, eng."=w544, "mmWave Axis Name"=w545, "UI MotionStatus in"=w546) -> ()  [unwired: 7 in, 2 out]
          }
          frame 1001 {
            # "motion started or stopped, mmWave"
            n281 = To Long Integer(number=w551) -> (32bit integer=w550:i32)
            n282 = Unbundle By Name(w554) -> ("MotionStatus"=w553:refnum<class "UI MotionStatus.lvclass">)
            n283 = Equal?(x=w550, y=1) -> (x = y?=w548:bool)
            n284 = call "WritemmWaveMoving.vi"("Axis Moving = True"=w548, "mmWave Axis Name"=w552, "UI MotionStatus in"=w553) -> ()  [unwired: 7 in, 2 out]
          }
        }
      }
      frame "AboutAPAR" {
        n285 = Format Into String(format string="APAR Test Main Version %s" ("message"), w555) -> (resulting string=w557:string)  [unwired: 2 in, 1 out]
        n286 = One Button Dialog(message=w557) -> ()  [unwired: 1 in, 1 out]
      }
      frame "Open" {
        # "comes from File>>Open menu"
        n287 = File Dialog(7:"Please select a file . . ." ("prompt")) -> (0:w559:errorcluster, 1:w560:bool, 3:w561:path)  [unwired: 6 in, 1 out]
        n288 = case shown="False" w560 {
          tunnel: w561 -> [_ w566]
          frame True {
          }
          frame False {
            n289 = Format Into String(format string="\"%s\"\n\n\nWhat a wonderful file selection. :-)", w566) -> (resulting string=w564:string)  [unwired: 2 in, 1 out]
            n290 = One Button Dialog(message=w564) -> ()  [unwired: 1 in, 1 out]
          }
        }
        n291 = Unbundle(w559) -> ()  [unwired: 3 out]
      }
      frame "ClearError" {
        n292 = call "ConvertTo(error).vi"("Message Payload"=w570) -> ("Message Payload error"=w569:errorcluster)  [unwired: 9 in, 1 out]
        n293 = Unbundle By Name(w569) -> ("code"=w568:i32, "source"=w567:string)
        n294 = case shown="1" w568 {
          tunnel: w567 -> [_ _]
          frame 0, Default {
          }
          frame 1 {
            # "could take error action here\nfor selected error codes, and\nignore all other codes"
          }
        }
      }
      frame "GenerateTestError" {
        n295 = call "ConvertTo(error).vi"("Message Payload"=w573) -> ("Message Payload error"=w572:errorcluster)  [unwired: 9 in, 1 out]
      }
      frame "---Copy This Frame---" {
        # "Duplicate this frame when creating new messages.  Change this comment in the duplicated frame to describe this message."
      }
      frame "ExitNow" {
        # "Write ini file\nOther cleanup tasks here"
        # "Release the message \nque reference"
        n296 = call "Fire User Event - ExitEventLoop.vi"("user event ExitEventLoop"=w576) -> ()  [unwired: 10 in, 1 out]
        n297 = Release Queue(queue=w578, error in (no error)=w580) -> ()  [unwired: 1 in, 3 out]
      }
    }
    n298 = call "SendErrorMessageToErrorLoop.vi"("Error Message que"=w228, "error in (no error)"=w233, "Loop Message que"=w232) -> ("error out"=w229:errorcluster)  [unwired: 8 in]
    "i main" <- w242
  }
  n299 = stacked-sequence {
    tunnel: w22 -> [w584]
    tunnel: [w582] -> w21
    tunnel: w11 -> [w581]
    tunnel: w16 -> [_]
    frame #0 {
      n300 = Unregister For Events(event registration refnum=w584) -> (error out=w583:errorcluster)  [unwired: 1 in]
      n301 = call "Destroy User Events - ExitMultiLoop.vi"("error in (no error)"=w583, "user event array"=w581) -> ("error out"=w582:errorcluster)  [unwired: 9 in]
    }
  }
  n302 = disable-structure "Conditional Disable Structure" shown="RUN_TIME_ENGINE==True" {
    disable-tunnel: w21 -> [_ _]
    frame condition #0 (active) {
    }
    frame condition #1 {
      # "close FP if this is an exe"
      n303 = Current VI's Path() -> (path=w589:path)
      n304 = Open VI Reference(vi path=w589) -> (vi reference=w585:refnum<vi>, error out=w588:errorcluster)  [unwired: 5 in]
      n305 = invoke on="Invoke Node" class="VI" method="FP.Close"(reference=w585, error in=w588) -> (reference out=w586:refnum<vi>, error out=w587:errorcluster)  [unwired: 1 in, 1 out]
      n306 = Close Reference(reference=w586, error in (no error)=w587) -> ()  [unwired: 1 out]
    }
  }
